vi "Send Return Value.vi"(8 "error in (no error)":errorcluster, 10 "Return Value":variant, 11 "Response in":refnum<class "Call.lvclass">) -> (0 "error out":errorcluster)   [LabVIEW 2013, in "JKI_Python_Bridge_for_LV.lvlib" / "Call.lvclass"]
uses:
  Call.lvclass
  Server/Type Definitions/Python Response - Cluster.ctl
  Call.lvclass/Call.ctl
  Server/Server.lvclass
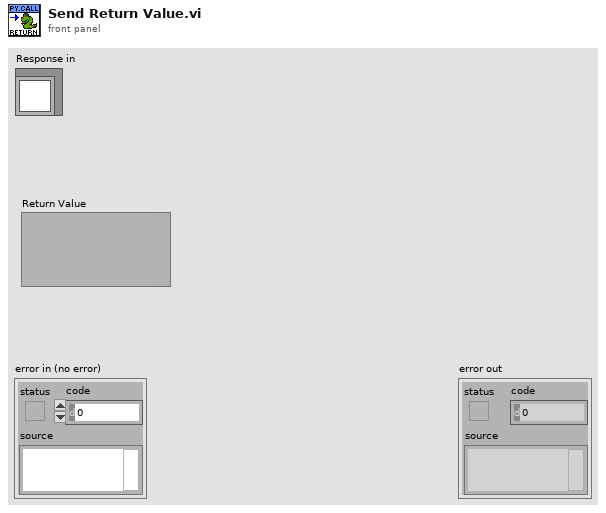
[diagram p1: front panel]
types:
  T1 = typedef "JKI_Python_Bridge_for_LV.lvlib/Server.lvclass/Python Response - Cluster.ctl" = cluster{"Python Response":variant, "error out":errorcluster}
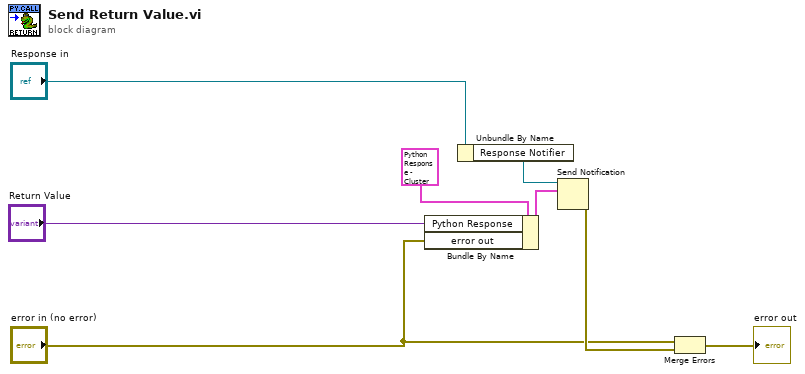
[diagram p0: block diagram]
diagram:
  n1 = Bundle By Name(cluster=T1 {"Python Response"=variant, "error out"={"status"=FALSE, "code"=0, "source"=""}} ("Python Response"), "Python Response"="Return Value", "error out"="error in (no error)") -> (w5:T1)
  n2 = Unbundle By Name("Response in") -> ("Response Notifier"=w7:refnum<notifier>)
  n3 = Send Notification(notification=w5, notifier=w7) -> (error out=w8:errorcluster)  [unwired: 1 in, 1 out]
  n4 = Merge Errors("error in (no error)", w8) -> (→"error out":errorcluster)
